vi "readMotor.vi"(0 "SPI Config In":T2) -> (1 "SPI Config Out":T2, 2 "Data Out":T1 {"ID" format="%x"})   [LabVIEW 2019]
uses:
  SPI/SPI Config.ctl
panel:
  in  "Data Out Reference":T1 {"ID" format="%x"}
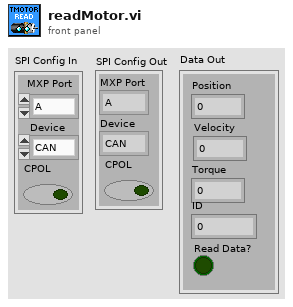
[diagram p1: front panel]
types:
  T1 = cluster{"Position":fxp<+/-,32,16>, "Velocity":fxp<+/-,32,16>, "Torque":fxp<+/-,32,16>, "ID":u32, "Read Data?":bool}
  T2 = typedef "SPI Config.ctl" = cluster{"MXP Port":enum16{"A", "B"}, "Device":enum16{"CAN", "ENC", "IMU1", "IMU2"}, "CPOL":bool}
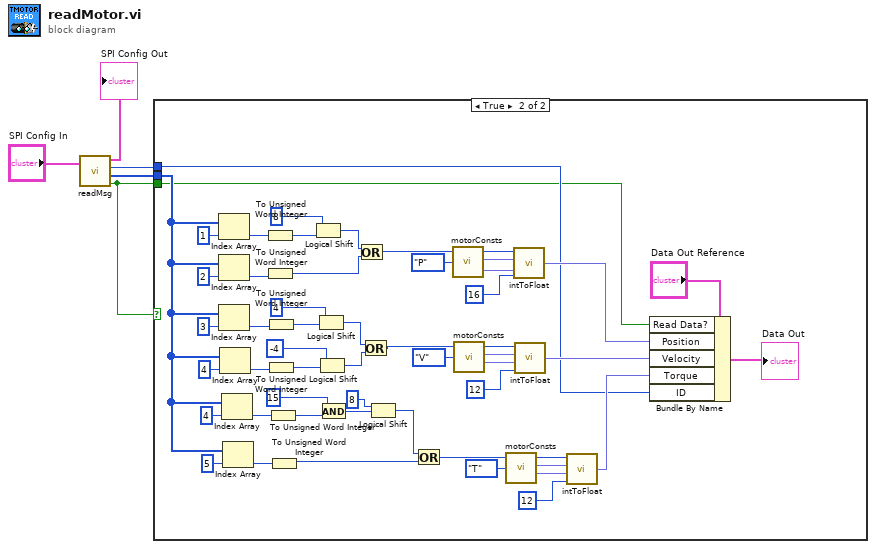
[diagram p0: block diagram]
diagram:
  n1 = call "readMsg.vi"("SPI Config In"="SPI Config In") -> ("SPI Config Out"=→"SPI Config Out":T2, "ID"=w4:u32, "CAN Msg"=w5:u8[], "Read Data?"=w1:bool)  [unwired: 1 in]
  n2 = case shown="True" w1 {
    tunnel: w5 -> [_ w15]
    tunnel: w4 -> [_ w9]
    tunnel: w1 -> [_ w6]
    frame False {
    }
    frame True {
      n3 = Index Array(array=w15, index=1) -> (element=w54:u8)
      n4 = Index Array(array=w15, index=2) -> (element=w53:u8)
      n5 = Index Array(array=w15, index=3) -> (element=w47:u8)
      n6 = Index Array(array=w15, index=4) -> (element=w43:u8)
      n7 = Index Array(array=w15, index=4) -> (element=w37:u8)
      n8 = Index Array(array=w15, index=5) -> (element=w31:u8)
      n9 = To Unsigned Word Integer(number=w54) -> (unsigned 16bit integer=w52:u16)
      n10 = To Unsigned Word Integer(number=w53) -> (unsigned 16bit integer=w49:u16)
      n11 = To Unsigned Word Integer(number=w47) -> (unsigned 16bit integer=w46:u16)
      n12 = To Unsigned Word Integer(number=w43) -> (unsigned 16bit integer=w42:u16)
      n13 = To Unsigned Word Integer(number=w37) -> (unsigned 16bit integer=w36:u16)
      n14 = To Unsigned Word Integer(number=w31) -> (unsigned 16bit integer=w29:u16)
      n15 = Logical Shift(y=i16 8, x=w52) -> (x << y=w50:u16)
      n16 = Logical Shift(y=i16 4, x=w46) -> (x << y=w40:u16)
      n17 = Logical Shift(y=i16 -4, x=w42) -> (x << y=w39:u16)
      n18 = And(x=u16 15, y=w36) -> (x .and. y?=w34:u16)
      n19 = Or(x=w50, y=w49) -> (x .or. y?=w28:u16)
      n20 = Or(x=w40, y=w39) -> (x .or. y?=w21:u16)
      n21 = Logical Shift(y=i16 8, x=w34) -> (x << y=w30:u16)
      n22 = Or(x=w30, y=w29) -> (x .or. y?=w16:u16)
      n23 = call "motorConsts.vi"("Parameter"=enum16{"P", "V", "T", "Kp", "Kd"}."P" ("Enum")) -> ("Max"=w14:fxp<+/-,32,16>, "Min"=w13:fxp<+/-,32,16>)
      n24 = call "motorConsts.vi"("Parameter"=enum16{"P", "V", "T", "Kp", "Kd"}."V" ("Enum")) -> ("Max"=w25:fxp<+/-,32,16>, "Min"=w24:fxp<+/-,32,16>)
      n25 = call "motorConsts.vi"("Parameter"=enum16{"P", "V", "T", "Kp", "Kd"}."T" ("Enum")) -> ("Max"=w20:fxp<+/-,32,16>, "Min"=w19:fxp<+/-,32,16>)
      n26 = call "intToFloat.vi"("bits"=i16 16, "x_min"=w13, "x_max"=w14, "x"=w28) -> ("Float"=w12:fxp<+/-,32,17>)
      n27 = call "intToFloat.vi"("bits"=i16 12, "x_min"=w24, "x_max"=w25, "x"=w21) -> ("Float"=w11:fxp<+/-,32,17>)
      n28 = call "intToFloat.vi"("bits"=i16 12, "x_min"=w19, "x_max"=w20, "x"=w16) -> ("Float"=w10:fxp<+/-,32,17>)
      n29 = Bundle By Name(cluster="Data Out Reference", "Read Data?"=w6, "Position"=w12, "Velocity"=w11, "Torque"=w10, "ID"=w9) -> (→"Data Out":T1)
    }
  }
